vi "NIVisOpenCV AprilTagdetection.vi"(5 "refine Edges":bool=TRUE, 6 "threads":i32=2, 7 "blur":dbl step=0.1, 8 "error in (no error)":errorcluster, 9 "decimate":dbl=2.0, 10 "Tag Familys":string[](array[combo])=["16h5"], 11 "Image Src":T2) -> (0 "error out":errorcluster, 2 "Detected Tags":T1(array[cluster]), 3 "Image Dst Out":T2, 4 "exec time (s)":dbl)   [LabVIEW 2023]
doc: "<b> NIVisOpenCV April Tag Detection</b> searches the image and describes tags in the Tag Familys. Parameters can be used to improve performance."
uses:
  <vilib>/vision/Image Controls.llb/IMAQ Image.ctl
  FRC_OpenCVExtensions.dll
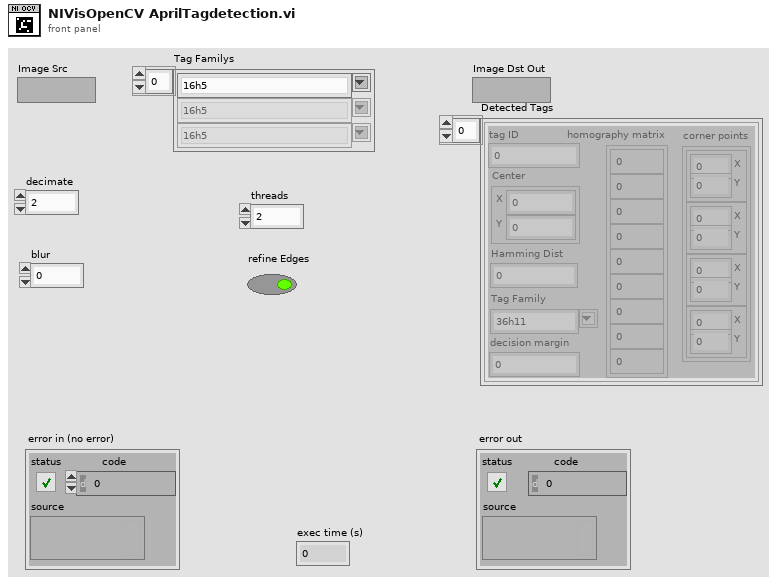
[diagram p1: front panel]
types:
  T1 = cluster{"tag ID":i32, "Center":cluster{"X":dbl, "Y":dbl}, "homography matrix":dbl[], "decision margin":dbl, "Hamming Dist":i32, "corner points":cluster{"X":dbl, "Y":dbl}[], "Tag Family":string}[]
  T2 = typedef "IMAQ Image.ctl" = refnum<image>
  T3 = cluster{"tag ID":i32, "Center":cluster{"X":dbl, "Y":dbl}, "Homography Matrix":dbl[], "dec margin":dbl, "Hamming Dist":i32, "Corner Points":cluster{"X":dbl, "Y":dbl}[], "familyID":i32}[]
  T4 = cluster{"tag ID":i32, "Center":cluster{"X":dbl, "Y":dbl}, "Homography Matrix":dbl[], "dec margin":dbl, "Hamming Dist":i32, "Corner Points":cluster{"X":dbl, "Y":dbl}[], "Tag Family":string}
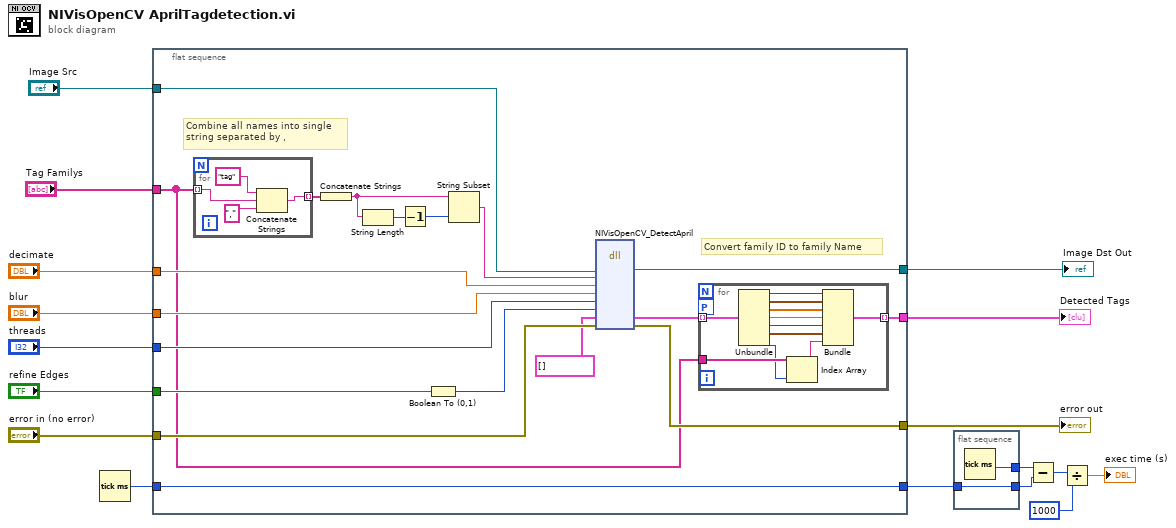
[diagram p0: block diagram]
diagram:
  n1 = Tick Count (ms)() -> (millisecond timer value=w7:u32)
  n2 = flat-sequence {
    tunnel: "Image Src" -> [w36]
    tunnel: [w35] -> w16
    tunnel: "decimate" -> [w34]
    tunnel: "blur" -> [w33]
    tunnel: "threads" -> [w32]
    tunnel: "refine Edges" -> [w31]
    tunnel: "error in (no error)" -> [w29]
    tunnel: [w28] -> w10
    tunnel: "Tag Familys" -> [w19]
    tunnel: [w25] -> w8
    tunnel: [w18] -> w6
    tunnel: w7 -> [w18]
    frame #0 {
      # "Convert family ID to family Name"
      # "Combine all names into single\nstring separated by ,"
      n3 = for {
        tunnel: w19 -> [w38] mode=indexing
        tunnel: [w39] -> w24 mode=indexing
        n4 = Concatenate Strings("tag" ("string"), w38, "," ("string")) -> (w39:string)
      }
      n5 = Concatenate Strings(w24) -> (w22:string)
      n6 = String Length(string=w22) -> (length=w21:i32)
      n7 = Decrement(x=w21) -> (x-1=w20:i32)
      n8 = Boolean To (0,1)(Boolean=w31) -> (0, 1=w30:i16)
      n9 = String Subset(string=w22, length (rest)=w20) -> (substring=w23:string)  [unwired: 1 in]
      n10 = dll-call lib="FRC_OpenCVExtensions.*" fn="NIVisOpenCV_DetectApril"("ImageA"=w36, "famName"=w23, "decimationValue"=w34, "blurValue"=w33, "workerThreads"=w32, "refineEdges"=w30, "ImageAPoints"=T3 [] ("Detected Tags"), "error"=w29) -> ("ImageA"=w35:T2, "ImageAPoints"=w26:T3, "error"=w28:errorcluster)  [unwired: 9 in, 2 out]
      n11 = for {
        tunnel: w26 -> [w51] mode=indexing
        tunnel: w19 -> [w44]
        tunnel: [w41] -> w25 mode=indexing
        workers-P: _ -> [_]
        n12 = Unbundle(w51) -> ("tag ID"=w50:i32, "Center"=w49:cluster{"X":dbl, "Y":dbl}, "Homography Matrix"=w48:dbl[], "dec margin"=w47:dbl, "Hamming Dist"=w46:i32, "Corner Points"=w45:cluster{"X":dbl, "Y":dbl}[], "familyID"=w43:i32)
        n13 = Index Array(array=w44, index=w43) -> (element=w42:string)
        n14 = Bundle("tag ID"=w50, "Center"=w49, "Homography Matrix"=w48, "dec margin"=w47, "Hamming Dist"=w46, "Corner Points"=w45, "Tag Family"=w42) -> (w41:T4)  [unwired: 1 in]
      }
    }
  }
  n15 = flat-sequence {
    tunnel: w6 -> [w52]
    tunnel: [w53] -> w5
    tunnel: [w52] -> w4
    frame #0 {
      n16 = Tick Count (ms)() -> (millisecond timer value=w53:u32)
    }
  }
  n17 = Subtract(x=w5, y=w4) -> (x-y=w3:u32)
  n18 = Divide(x=w3, y=u32 1000) -> (x/y=→"exec time (s)":dbl)
  "error out" <- w10
  "Image Dst Out" <- w16
  "Detected Tags" <- w8
